vi "Create 8 Out Channel Resources.vi"(0 "common resources":T8={"sync pulse resources"={"sync pulse destination terminal"="", "sync100"="", "sync pulse source terminal"="", "imported sync pulse register"="", "generate sync pulse handshake"="", "enable sync pulse register"="", "sync pulse clock"=""}, "serial channel resources"={"sc 0"={"completed frames register"=""}, "sc 1"={"completed frames register"=""}, "sc 2"={"completed frames register"=""}, "sc 3"={"completed frames register"=""}, "sc 4"={"completed frames register"=""}, "sc 5"={"completed frames register"=""}, "sc 6"={"completed frames register"=""}, "sc 7"={"completed frames register"=""}}, "dram manager 0"={"DRAM class"=refnum, "process clock"="", "registers"={"configuration"={"write time slice"="", "request time slice"="", "DRAM arbiter config"="", "partition config"=""}, "reset"={"handshake"={"start.go"="", "start.go rcvd"="", "done.go"="", "done.go rcvd"=""}, "process"={"in"="", "out"=""}, "write"={"in"="", "out 0"="", "out 1"="", "out 2"="", "out 3"=""}, "read"={"in"="", "out 0"="", "out 1"="", "out 2"="", "out 3"=""}}, "status"={"partition full"=""}}, "FIFOs"={"write data"={"FIFO 0"="", "FIFO 1"="", "FIFO 2"="", "FIFO 3"=""}, "request metadata"={"FIFO"=""}, "read data VOQ"={"FIFO 0"="", "FIFO 1"="", "FIFO 2"="", "FIFO 3"=""}, "read data"={"FIFO 0"="", "FIFO 1"="", "FIFO 2"="", "FIFO 3"=""}}, "num active streams"=0.0, "max open read requests"=256}, "dram manager 1"={"DRAM class"=refnum, "process clock"="", "registers"={"configuration"={"write time slice"="", "request time slice"="", "DRAM arbiter config"="", "partition config"=""}, "reset"={"handshake"={"start.go"="", "start.go rcvd"="", "done.go"="", "done.go rcvd"=""}, "process"={"in"="", "out"=""}, "write"={"in"="", "out 0"="", "out 1"="", "out 2"="", "out 3"=""}, "read"={"in"="", "out 0"="", "out 1"="", "out 2"="", "out 3"=""}}, "status"={"partition full"=""}}, "FIFOs"={"write data"={"FIFO 0"="", "FIFO 1"="", "FIFO 2"="", "FIFO 3"=""}, "request metadata"={"FIFO"=""}, "read data VOQ"={"FIFO 0"="", "FIFO 1"="", "FIFO 2"="", "FIFO 3"=""}, "read data"={"FIFO 0"="", "FIFO 1"="", "FIFO 2"="", "FIFO 3"=""}}, "num active streams"=0.0, "max open read requests"=256}}) -> (4 "channel resources":T1)   [LabVIEW 2020, in "GettingStarted_Gen_148X_FPGA.lvlib"]
uses:
  GettingStarted_Gen_148X_FPGA.lvlib
  Common/Types/Common Resources.ctl
  <instrlib>/_niInstr/Memory/v1/FPGA/DRAM/niInstr Memory DRAM v1 FPGA.lvclass
  <instrlib>/FlexRIO/CSI-2/v2/FPGA/Types/Sync Pulse Resources.ctl
  Common/Types/Serial Channel Resources.ctl
  Common/Types/Single Serial Channel Resources.ctl
  <instrlib>/FlexRIO/CSI-2/v2/FPGA/DRAM Manager/Private/DRAM Manager.ctl
  <instrlib>/FlexRIO/CSI-2/v2/FPGA/DRAM Manager/Private/Common/DRAM Manager Registers.ctl
  <instrlib>/FlexRIO/CSI-2/v2/FPGA/DRAM Manager/Private/Common/Handshake Registers.ctl
  <instrlib>/FlexRIO/CSI-2/v2/FPGA/DRAM Manager/Private/Common/DRAM Manager FIFOs.ctl
  <instrlib>/FlexRIO/CSI-2/v2/FPGA/DRAM Manager/Private/Common/Write Data FIFO Ref.ctl
  <instrlib>/FlexRIO/CSI-2/v2/FPGA/DRAM Manager/Private/Common/Read Request Metadata FIFO Ref.ctl
  <instrlib>/FlexRIO/CSI-2/v2/FPGA/DRAM Manager/Private/Common/Read Data FIFO Ref.ctl
  Types/8 Out Channel Resources.ctl
  Types/Serial Output Channel Resources.ctl
  Common/Types/Serial Output Channel IO.ctl
  Common/Types/Serial Output Channel IO 32b.ctl
  Common/Types/Serial Output Channel IO 64b.ctl
  Common/Types/I2C IO.ctl
  Common/GettingStarted_Common_148X_FPGA.lvlib
  <instrlib>/FlexRIO/CSI-2/v2/FPGA/DRAM Manager/DRAM Manager v2.lvlib
  <instrlib>/FlexRIO/CSI-2/v2/FPGA/NI CSI-2 API FPGA v2.lvlib
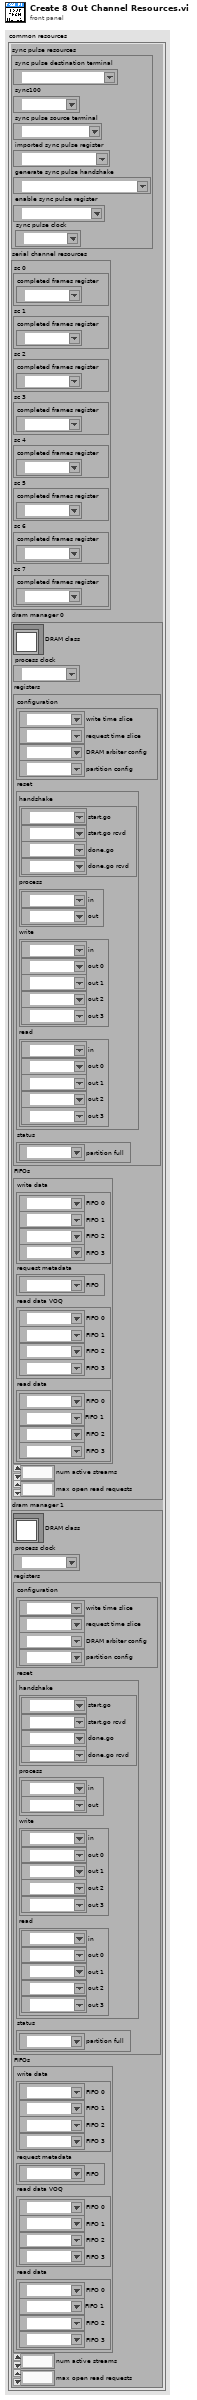
[diagram p1: front panel]
types:
  T1 = typedef "GettingStarted_Gen_148X_FPGA.lvlib/8 Out Channel Resources.ctl" = cluster{"so 0 resources":T2, "so 1 resources":T2, "so 2 resources":T2, "so 3 resources":T2, "so 4 resources":T2, "so 5 resources":T2, "so 6 resources":T2, "so 7 resources":T2}
  T2 = typedef "GettingStarted_Gen_148X_FPGA.lvlib/Serial Output Channel Resources.ctl" = cluster{"csi-2 output io":T3, "serial output channel instance":u8, "i2c io":T6, "sc resources":T7}
  T3 = typedef "GettingStarted_Common_148X_FPGA.lvlib/Serial Output Channel IO.ctl" = cluster{"32b":T4, "64b":T5, "csi-2 axi stream tready":refnum<k21>, "csi-2 axi stream tvalid":refnum<k21>, "csi-2 axi stream tlast":refnum<k21>, "num packets in tx fifo":refnum<k21>, "ready to transmit packet":refnum<k21>, "transmit packet done":refnum<k21>, "transmit packet":refnum<k21>}
  T4 = typedef "GettingStarted_Common_148X_FPGA.lvlib/Serial Output Channel IO 32b.ctl" = cluster{"csi-2 axi stream tdata":refnum<k21>, "csi-2 axi stream tuser":refnum<k21>}
  T5 = typedef "GettingStarted_Common_148X_FPGA.lvlib/Serial Output Channel IO 64b.ctl" = cluster{"csi-2 axi stream tdata":refnum<k21>, "csi-2 axi stream tuser":refnum<k21>}
  T6 = typedef "GettingStarted_Common_148X_FPGA.lvlib/I2C IO.ctl" = cluster{"sda input":refnum<k21>, "sda output enable":refnum<k21>, "scl input":refnum<k21>, "scl output enable":refnum<k21>}
  T7 = typedef "GettingStarted_Common_148X_FPGA.lvlib/Single Serial Channel Resources.ctl" = cluster{"completed frames register":refnum<k21>}
  T8 = typedef "GettingStarted_Common_148X_FPGA.lvlib/Common Resources.ctl" = cluster{"sync pulse resources":T9, "serial channel resources":T10, "dram manager 0":T11, "dram manager 1":T11}
  T9 = typedef "NI CSI-2 API FPGA v2.lvlib/Sync Pulse Resources.ctl" = cluster{"sync pulse destination terminal":refnum<k21>, "sync100":refnum<k21>, "sync pulse source terminal":refnum<k21>, "imported sync pulse register":refnum<k21>, "generate sync pulse handshake":refnum<k21>, "enable sync pulse register":refnum<k21>, "sync pulse clock":refnum<k21>}
  T10 = typedef "GettingStarted_Common_148X_FPGA.lvlib/Serial Channel Resources.ctl" = cluster{"sc 0":T7, "sc 1":T7, "sc 2":T7, "sc 3":T7, "sc 4":T7, "sc 5":T7, "sc 6":T7, "sc 7":T7}
  T11 = typedef "DRAM Manager v2.lvlib/DRAM Manager.ctl" = cluster{"DRAM class":refnum<class "niInstr Memory DRAM v1 FPGA.lvclass">, "process clock":refnum<k21>, "registers":T12, "FIFOs":T14, "num active streams":fxp<+,3,3>, "max open read requests":u16}
  T12 = typedef "DRAM Manager v2.lvlib/DRAM Manager Registers.ctl" = cluster{"configuration":cluster{"write time slice":refnum<k21>, "request time slice":refnum<k21>, "DRAM arbiter config":refnum<k21>, "partition config":refnum<k21>}, "reset":cluster{"handshake":T13, "process":cluster{"in":refnum<k21>, "out":refnum<k21>}, "write":cluster{"in":refnum<k21>, "out 0":refnum<k21>, "out 1":refnum<k21>, "out 2":refnum<k21>, "out 3":refnum<k21>}, "read":cluster{"in":refnum<k21>, "out 0":refnum<k21>, "out 1":refnum<k21>, "out 2":refnum<k21>, "out 3":refnum<k21>}}, "status":cluster{"partition full":refnum<k21>}}
  T13 = typedef "DRAM Manager v2.lvlib/Handshake Registers.ctl" = cluster{"start.go":refnum<k21>, "start.go rcvd":refnum<k21>, "done.go":refnum<k21>, "done.go rcvd":refnum<k21>}
  T14 = typedef "DRAM Manager v2.lvlib/DRAM Manager FIFOs.ctl" = cluster{"write data":cluster{"FIFO 0":T15, "FIFO 1":T15, "FIFO 2":T15, "FIFO 3":T15}, "request metadata":cluster{"FIFO":T16}, "read data VOQ":cluster{"FIFO 0":T17, "FIFO 1":T17, "FIFO 2":T17, "FIFO 3":T17}, "read data":cluster{"FIFO 0":T17, "FIFO 1":T17, "FIFO 2":T17, "FIFO 3":T17}}
  T15 = typedef "DRAM Manager v2.lvlib/Write Data FIFO Ref.ctl" = refnum<k21>
  T16 = typedef "DRAM Manager v2.lvlib/Read Request Metadata FIFO Ref.ctl" = refnum<k21>
  T17 = typedef "DRAM Manager v2.lvlib/Read Data FIFO Ref.ctl" = refnum<k21>
  T18 = cluster{"serial output 0 csi-2 io":T3, "serial output 1 csi-2 io":T3, "serial output 2 csi-2 io":T3, "serial output 3 csi-2 io":T3, "serial output 4 csi-2 io":T3, "serial output 5 csi-2 io":T3, "serial output 6 csi-2 io":T3, "serial output 7 csi-2 io":T3}
  T19 = cluster{"serial output 2 i2c io":T6, "serial output 1 i2c io":T6, "serial output 0 i2c io":T6, "serial output 3 i2c io":T6, "serial output 4 i2c io":T6, "serial output 5 i2c io":T6, "serial output 6 i2c io":T6, "serial output 7 i2c io":T6}
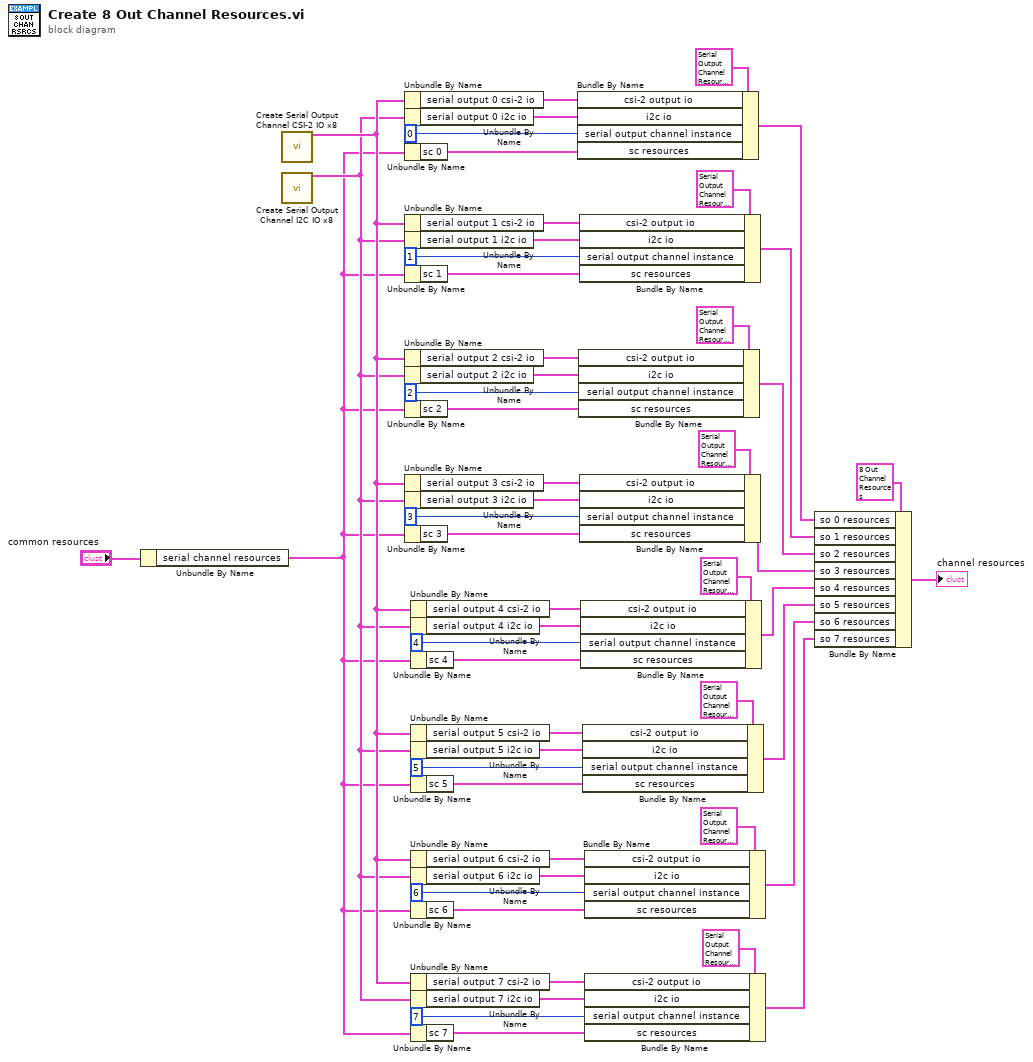
[diagram p0: block diagram]
diagram:
  n1 = Unbundle By Name("common resources") -> ("serial channel resources"=w9:T10)
  n2 = call "Create Serial Output Channel CSI-2 IO x8.vi"() -> ("serial output channel io x8"=w19:T18)  [unwired: 15 in]
  n3 = call "Create Serial Output Channel I2C IO x8.vi"() -> ("serial output channel i2c io x8"=w18:T19)  [unwired: 15 in]
  n4 = Unbundle By Name(w19) -> ("serial output 0 csi-2 io"=w22:T3)
  n5 = Unbundle By Name(w18) -> ("serial output 0 i2c io"=w37:T6)
  n6 = Unbundle By Name(w9) -> ("sc 0"=w8:T7)
  n7 = Unbundle By Name(w19) -> ("serial output 1 csi-2 io"=w36:T3)
  n8 = Unbundle By Name(w18) -> ("serial output 1 i2c io"=w35:T6)
  n9 = Unbundle By Name(w9) -> ("sc 1"=w7:T7)
  n10 = Unbundle By Name(w19) -> ("serial output 2 csi-2 io"=w34:T3)
  n11 = Unbundle By Name(w18) -> ("serial output 2 i2c io"=w33:T6)
  n12 = Unbundle By Name(w9) -> ("sc 2"=w6:T7)
  n13 = Unbundle By Name(w19) -> ("serial output 3 csi-2 io"=w32:T3)
  n14 = Unbundle By Name(w18) -> ("serial output 3 i2c io"=w31:T6)
  n15 = Unbundle By Name(w9) -> ("sc 3"=w5:T7)
  n16 = Unbundle By Name(w19) -> ("serial output 4 csi-2 io"=w30:T3)
  n17 = Unbundle By Name(w18) -> ("serial output 4 i2c io"=w29:T6)
  n18 = Unbundle By Name(w9) -> ("sc 4"=w4:T7)
  n19 = Unbundle By Name(w19) -> ("serial output 5 csi-2 io"=w28:T3)
  n20 = Unbundle By Name(w18) -> ("serial output 5 i2c io"=w27:T6)
  n21 = Unbundle By Name(w9) -> ("sc 5"=w1:T7)
  n22 = Unbundle By Name(w19) -> ("serial output 6 csi-2 io"=w26:T3)
  n23 = Unbundle By Name(w18) -> ("serial output 6 i2c io"=w25:T6)
  n24 = Unbundle By Name(w9) -> ("sc 6"=w3:T7)
  n25 = Unbundle By Name(w19) -> ("serial output 7 csi-2 io"=w24:T3)
  n26 = Unbundle By Name(w18) -> ("serial output 7 i2c io"=w23:T6)
  n27 = Unbundle By Name(w9) -> ("sc 7"=w2:T7)
  n28 = Bundle By Name(cluster=T2 {"csi-2 output io"={"32b"={"csi-2 axi stream tdata"="", "csi-2 axi stream tuser"=""}, "64b"={"csi-2 axi stream tdata"="", "csi-2 axi stream tuser"=""}, "csi-2 axi stream tready"="", "csi-2 axi stream tvalid"="", "csi-2 axi stream tlast"="", "num packets in tx fifo"="", "ready to transmit packet"="", "transmit packet done"="", "transmit packet"=""}, "serial output channel instance"=0, "i2c io"={"sda input"="", "sda output enable"="", "scl input"="", "scl output enable"=""}, "sc resources"={"completed frames register"=""}} ("si 0 resources"), "csi-2 output io"=w22, "i2c io"=w37, "serial output channel instance"=u8 0 ("serial input channel instance"), "sc resources"=w8) -> (w52:T2)
  n29 = Bundle By Name(cluster=T2 {"csi-2 output io"={"32b"={"csi-2 axi stream tdata"="", "csi-2 axi stream tuser"=""}, "64b"={"csi-2 axi stream tdata"="", "csi-2 axi stream tuser"=""}, "csi-2 axi stream tready"="", "csi-2 axi stream tvalid"="", "csi-2 axi stream tlast"="", "num packets in tx fifo"="", "ready to transmit packet"="", "transmit packet done"="", "transmit packet"=""}, "serial output channel instance"=0, "i2c io"={"sda input"="", "sda output enable"="", "scl input"="", "scl output enable"=""}, "sc resources"={"completed frames register"=""}} ("si 0 resources"), "csi-2 output io"=w34, "i2c io"=w33, "serial output channel instance"=u8 2 ("serial input channel instance"), "sc resources"=w6) -> (w48:T2)
  n30 = Bundle By Name(cluster=T2 {"csi-2 output io"={"32b"={"csi-2 axi stream tdata"="", "csi-2 axi stream tuser"=""}, "64b"={"csi-2 axi stream tdata"="", "csi-2 axi stream tuser"=""}, "csi-2 axi stream tready"="", "csi-2 axi stream tvalid"="", "csi-2 axi stream tlast"="", "num packets in tx fifo"="", "ready to transmit packet"="", "transmit packet done"="", "transmit packet"=""}, "serial output channel instance"=0, "i2c io"={"sda input"="", "sda output enable"="", "scl input"="", "scl output enable"=""}, "sc resources"={"completed frames register"=""}} ("si 0 resources"), "csi-2 output io"=w36, "i2c io"=w35, "serial output channel instance"=u8 1 ("serial input channel instance"), "sc resources"=w7) -> (w50:T2)
  n31 = Bundle By Name(cluster=T2 {"csi-2 output io"={"32b"={"csi-2 axi stream tdata"="", "csi-2 axi stream tuser"=""}, "64b"={"csi-2 axi stream tdata"="", "csi-2 axi stream tuser"=""}, "csi-2 axi stream tready"="", "csi-2 axi stream tvalid"="", "csi-2 axi stream tlast"="", "num packets in tx fifo"="", "ready to transmit packet"="", "transmit packet done"="", "transmit packet"=""}, "serial output channel instance"=0, "i2c io"={"sda input"="", "sda output enable"="", "scl input"="", "scl output enable"=""}, "sc resources"={"completed frames register"=""}} ("si 0 resources"), "csi-2 output io"=w32, "i2c io"=w31, "serial output channel instance"=u8 3 ("serial input channel instance"), "sc resources"=w5) -> (w46:T2)
  n32 = Bundle By Name(cluster=T2 {"csi-2 output io"={"32b"={"csi-2 axi stream tdata"="", "csi-2 axi stream tuser"=""}, "64b"={"csi-2 axi stream tdata"="", "csi-2 axi stream tuser"=""}, "csi-2 axi stream tready"="", "csi-2 axi stream tvalid"="", "csi-2 axi stream tlast"="", "num packets in tx fifo"="", "ready to transmit packet"="", "transmit packet done"="", "transmit packet"=""}, "serial output channel instance"=0, "i2c io"={"sda input"="", "sda output enable"="", "scl input"="", "scl output enable"=""}, "sc resources"={"completed frames register"=""}} ("si 0 resources"), "csi-2 output io"=w30, "i2c io"=w29, "serial output channel instance"=u8 4 ("serial input channel instance"), "sc resources"=w4) -> (w44:T2)
  n33 = Bundle By Name(cluster=T2 {"csi-2 output io"={"32b"={"csi-2 axi stream tdata"="", "csi-2 axi stream tuser"=""}, "64b"={"csi-2 axi stream tdata"="", "csi-2 axi stream tuser"=""}, "csi-2 axi stream tready"="", "csi-2 axi stream tvalid"="", "csi-2 axi stream tlast"="", "num packets in tx fifo"="", "ready to transmit packet"="", "transmit packet done"="", "transmit packet"=""}, "serial output channel instance"=0, "i2c io"={"sda input"="", "sda output enable"="", "scl input"="", "scl output enable"=""}, "sc resources"={"completed frames register"=""}} ("si 0 resources"), "csi-2 output io"=w28, "i2c io"=w27, "serial output channel instance"=u8 5 ("serial input channel instance"), "sc resources"=w1) -> (w42:T2)
  n34 = Bundle By Name(cluster=T2 {"csi-2 output io"={"32b"={"csi-2 axi stream tdata"="", "csi-2 axi stream tuser"=""}, "64b"={"csi-2 axi stream tdata"="", "csi-2 axi stream tuser"=""}, "csi-2 axi stream tready"="", "csi-2 axi stream tvalid"="", "csi-2 axi stream tlast"="", "num packets in tx fifo"="", "ready to transmit packet"="", "transmit packet done"="", "transmit packet"=""}, "serial output channel instance"=0, "i2c io"={"sda input"="", "sda output enable"="", "scl input"="", "scl output enable"=""}, "sc resources"={"completed frames register"=""}} ("si 0 resources"), "csi-2 output io"=w26, "i2c io"=w25, "serial output channel instance"=u8 6 ("serial input channel instance"), "sc resources"=w3) -> (w40:T2)
  n35 = Bundle By Name(cluster=T2 {"csi-2 output io"={"32b"={"csi-2 axi stream tdata"="", "csi-2 axi stream tuser"=""}, "64b"={"csi-2 axi stream tdata"="", "csi-2 axi stream tuser"=""}, "csi-2 axi stream tready"="", "csi-2 axi stream tvalid"="", "csi-2 axi stream tlast"="", "num packets in tx fifo"="", "ready to transmit packet"="", "transmit packet done"="", "transmit packet"=""}, "serial output channel instance"=0, "i2c io"={"sda input"="", "sda output enable"="", "scl input"="", "scl output enable"=""}, "sc resources"={"completed frames register"=""}} ("si 0 resources"), "csi-2 output io"=w24, "i2c io"=w23, "serial output channel instance"=u8 7 ("serial input channel instance"), "sc resources"=w2) -> (w38:T2)
  n36 = Bundle By Name(cluster=T1 {"so 0 resources"={"csi-2 output io"={"32b"={"csi-2 axi stream tdata"="", "csi-2 axi stream tuser"=""}, "64b"={"csi-2 axi stream tdata"="", "csi-2 axi stream tuser"=""}, "csi-2 axi stream tready"="", "csi-2 axi stream tvalid"="", "csi-2 axi stream tlast"="", "num packets in tx fifo"="", "ready to transmit packet"="", "transmit packet done"="", "transmit packet"=""}, "serial output channel instance"=0, "i2c io"={"sda input"="", "sda output enable"="", "scl input"="", "scl output enable"=""}, "sc resources"={"completed frames register"=""}}, "so 1 resources"={"csi-2 output io"={"32b"={"csi-2 axi stream tdata"="", "csi-2 axi stream tuser"=""}, "64b"={"csi-2 axi stream tdata"="", "csi-2 axi stream tuser"=""}, "csi-2 axi stream tready"="", "csi-2 axi stream tvalid"="", "csi-2 axi stream tlast"="", "num packets in tx fifo"="", "ready to transmit packet"="", "transmit packet done"="", "transmit packet"=""}, "serial output channel instance"=0, "i2c io"={"sda input"="", "sda output enable"="", "scl input"="", "scl output enable"=""}, "sc resources"={"completed frames register"=""}}, "so 2 resources"={"csi-2 output io"={"32b"={"csi-2 axi stream tdata"="", "csi-2 axi stream tuser"=""}, "64b"={"csi-2 axi stream tdata"="", "csi-2 axi stream tuser"=""}, "csi-2 axi stream tready"="", "csi-2 axi stream tvalid"="", "csi-2 axi stream tlast"="", "num packets in tx fifo"="", "ready to transmit packet"="", "transmit packet done"="", "transmit packet"=""}, "serial output channel instance"=0, "i2c io"={"sda input"="", "sda output enable"="", "scl input"="", "scl output enable"=""}, "sc resources"={"completed frames register"=""}}, "so 3 resources"={"csi-2 output io"={"32b"={"csi-2 axi stream tdata"="", "csi-2 axi stream tuser"=""}, "64b"={"csi-2 axi stream tdata"="", "csi-2 axi stream tuser"=""}, "csi-2 axi stream tready"="", "csi-2 axi stream tvalid"="", "csi-2 axi stream tlast"="", "num packets in tx fifo"="", "ready to transmit packet"="", "transmit packet done"="", "transmit packet"=""}, "serial output channel instance"=0, "i2c io"={"sda input"="", "sda output enable"="", "scl input"="", "scl output enable"=""}, "sc resources"={"completed frames register"=""}}, "so 4 resources"={"csi-2 output io"={"32b"={"csi-2 axi stream tdata"="", "csi-2 axi stream tuser"=""}, "64b"={"csi-2 axi stream tdata"="", "csi-2 axi stream tuser"=""}, "csi-2 axi stream tready"="", "csi-2 axi stream tvalid"="", "csi-2 axi stream tlast"="", "num packets in tx fifo"="", "ready to transmit packet"="", "transmit packet done"="", "transmit packet"=""}, "serial output channel instance"=0, "i2c io"={"sda input"="", "sda output enable"="", "scl input"="", "scl output enable"=""}, "sc resources"={"completed frames register"=""}}, "so 5 resources"={"csi-2 output io"={"32b"={"csi-2 axi stream tdata"="", "csi-2 axi stream tuser"=""}, "64b"={"csi-2 axi stream tdata"="", "csi-2 axi stream tuser"=""}, "csi-2 axi stream tready"="", "csi-2 axi stream tvalid"="", "csi-2 axi stream tlast"="", "num packets in tx fifo"="", "ready to transmit packet"="", "transmit packet done"="", "transmit packet"=""}, "serial output channel instance"=0, "i2c io"={"sda input"="", "sda output enable"="", "scl input"="", "scl output enable"=""}, "sc resources"={"completed frames register"=""}}, "so 6 resources"={"csi-2 output io"={"32b"={"csi-2 axi stream tdata"="", "csi-2 axi stream tuser"=""}, "64b"={"csi-2 axi stream tdata"="", "csi-2 axi stream tuser"=""}, "csi-2 axi stream tready"="", "csi-2 axi stream tvalid"="", "csi-2 axi stream tlast"="", "num packets in tx fifo"="", "ready to transmit packet"="", "transmit packet done"="", "transmit packet"=""}, "serial output channel instance"=0, "i2c io"={"sda input"="", "sda output enable"="", "scl input"="", "scl output enable"=""}, "sc resources"={"completed frames register"=""}}, "so 7 resources"={"csi-2 output io"={"32b"={"csi-2 axi stream tdata"="", "csi-2 axi stream tuser"=""}, "64b"={"csi-2 axi stream tdata"="", "csi-2 axi stream tuser"=""}, "csi-2 axi stream tready"="", "csi-2 axi stream tvalid"="", "csi-2 axi stream tlast"="", "num packets in tx fifo"="", "ready to transmit packet"="", "transmit packet done"="", "transmit packet"=""}, "serial output channel instance"=0, "i2c io"={"sda input"="", "sda output enable"="", "scl input"="", "scl output enable"=""}, "sc resources"={"completed frames register"=""}}}, "so 0 resources"=w52, "so 1 resources"=w50, "so 2 resources"=w48, "so 3 resources"=w46, "so 4 resources"=w44, "so 5 resources"=w42, "so 6 resources"=w40, "so 7 resources"=w38) -> (→"channel resources":T1)
